vi "Update route + target location.vi"(9 "Route":dbl[][](array[numeric]), 10 "Map input":dbl[][](array[numeric]), 11 "Target Location":dbl[](array[numeric])) -> (3 "Map Output":dbl[][](array[numeric]))   [LabVIEW 2015]
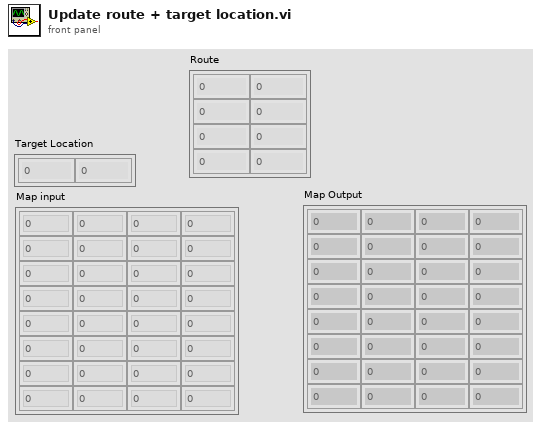
[diagram p1: front panel]
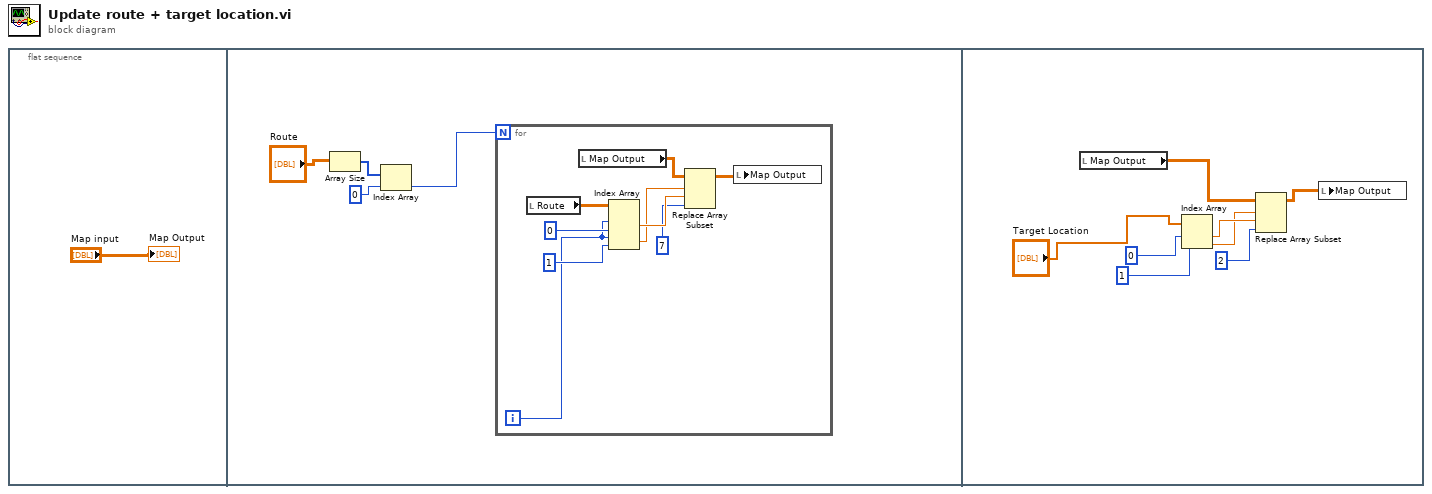
[diagram p0: block diagram]
diagram:
  n1 = flat-sequence {
    frame #0 {
      "Map Output" <- "Map input"
    }
    frame #1 {
      n2 = Array Size(array="Route") -> (size(s)=w4:i32[])
      n3 = Index Array(array=w4, index=0) -> (element=w2:i32)
      n4 = for {
        N: w2 -> [_]
        i -> [w6]
        n5 = local read "Route"() -> (w14:dbl[][])
        n6 = local read "Map Output"() -> (w13:dbl[][])
        n7 = Index Array(array=w14, index (row) #1=w6, index (col) #1=0, index (row) #2=w6, index (col) #2=1) -> (element #1=w11:dbl, element #2=w10:dbl)
        n8 = Replace Array Subset(array=w13, new element=7, index (row)=w10, index (col)=w11) -> (w12:dbl[][])
        n9 = local write "Map Output"(w12) -> ()
      }
    }
    frame #2 {
      n10 = local read "Map Output"() -> (w20:dbl[][])
      n11 = Index Array(array="Target Location", index #1=0, index #2=1) -> (element #1=w19:dbl, element #2=w15:dbl)
      n12 = Replace Array Subset(array=w20, new element=2, index (row)=w15, index (col)=w19) -> (w21:dbl[][])
      n13 = local write "Map Output"(w21) -> ()
    }
  }
